vi "TestLightfield.vi"() -> ()   [LabVIEW 2018]
uses:
  <userlib>/LightField Add-in and Automation SDK/Samples/LabVIEW Automation/lightfield-automation-labview/LightField Automation.lvclass
panel:
  out "LightField Error":errorcluster
  in  "Number of Frames":i32=500 min=0 step=1
  in  "On Chip Accumulations":i32=3 min=0 step=1
  in  "stop":bool
  in  "LIGHTFIELD":bool
  in  "Intensifier Gain":i32=100 min=0 max=100 step=1
  in  "Repetitive Gate Delay (us)":dbl=0.25
  in  "Repetitive Gate Width (us)":dbl=400.0 min=0.0 step=0.0001
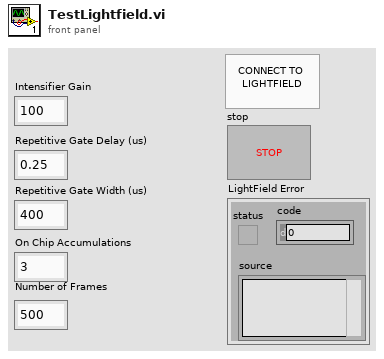
[diagram p1: front panel]
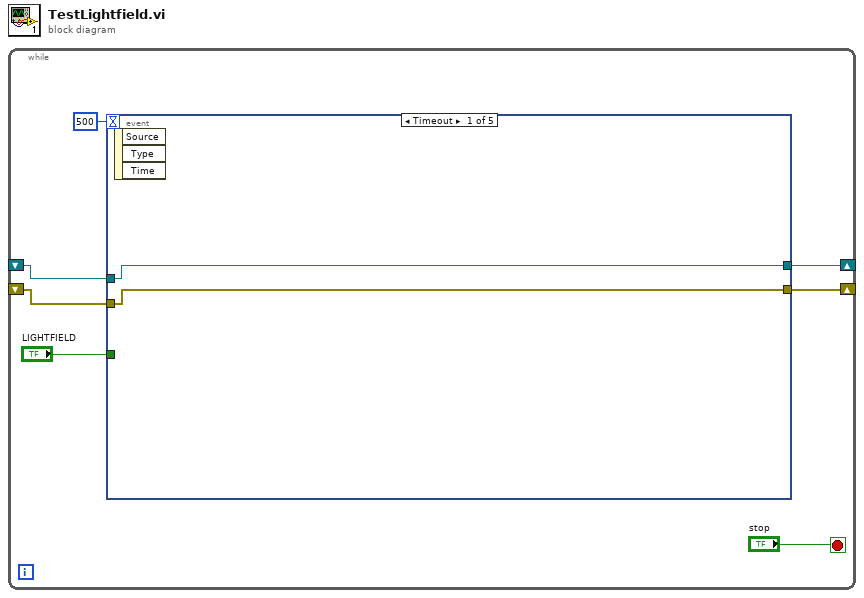
[diagram p0: block diagram]
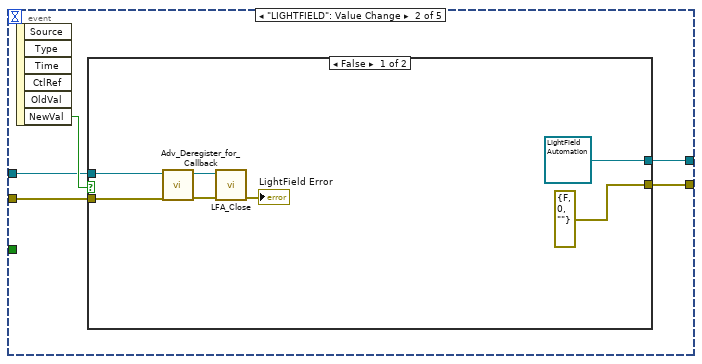
[diagram p2: hidden frame]
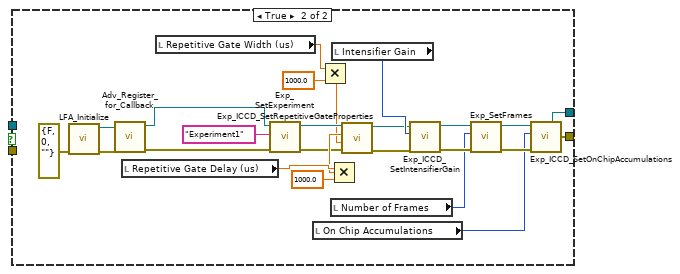
[diagram p3: hidden frame]
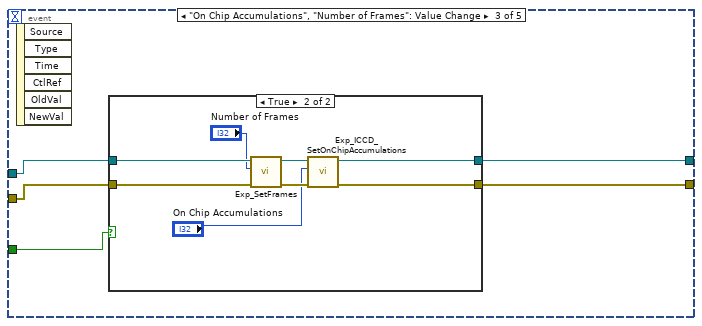
[diagram p4: hidden frame]
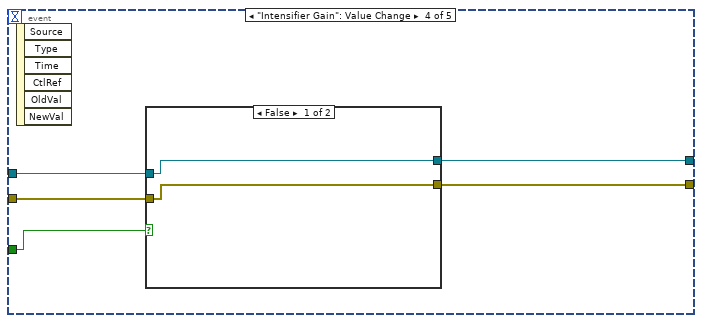
[diagram p6: hidden frame]
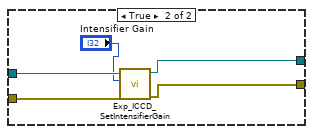
[diagram p7: hidden frame]
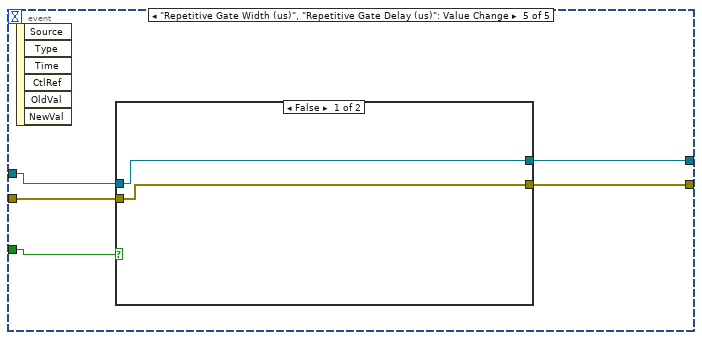
[diagram p8: hidden frame]
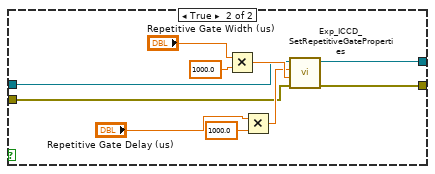
[diagram p9: hidden frame]
diagram:
  n1 = while {
    shift-right: [w4] -> _
    shift-left: _ -> [w7]
    shift-right: [w5] -> _
    shift-left: _ -> [w6]
    stop <- "stop" stop-if-true
    n2 = event shown="[0] Timeout" {
      selector: _ -> [_ _ _ _ _]
      dyn-events: _ -> [_ _ _ _ _]
      timeout: 500 -> [_ _ _ _ _]
      tunnel: w7 -> [w9 w13 w50 w66 w77]
      tunnel: w6 -> [w8 w12 w51 w65 w78]
      tunnel: [w8 w11 w48 w63 w75] -> w5
      tunnel: [w9 w10 w49 w64 w76] -> w4
      tunnel: "LIGHTFIELD" -> [_ _ w47 w62 w74]
      event Timeout {
        n3 = event-data() -> ()  [unwired: 1 in, 3 out]
      }
      event "LIGHTFIELD": Value Change {
        n4 = event-data() -> ("NewVal"=w14:bool)  [unwired: 1 in, 5 out]
        n5 = case shown="False" w14 {
          tunnel: w13 -> [w17 _]
          tunnel: w12 -> [w18 _]
          tunnel: [errorcluster {"status"=FALSE, "code"=0, "source"=""} ("error out") w28] -> w11
          tunnel: [refnum<class "LightField Automation.lvclass"> refnum ("LightField Automation out") w27] -> w10
          frame False {
            n6 = call <userlib>:"Adv_Deregister_for_Callback.vi"("error in (no error)"=w18, "LightField Automation in"=w17) -> ("error out"=w20:errorcluster, "LightField Automation out"=w19:refnum<class "LightField Automation.lvclass">)  [unwired: 8 in]
            n7 = call <userlib>:"LFA_Close.vi"("error in (no error)"=w20, "LightField Automation in"=w19) -> ("error out"=→"LightField Error":errorcluster)  [unwired: 8 in, 1 out]
          }
          frame True {
            n8 = call <userlib>:"LFA_Initialize.vi"("error in (no error)"=errorcluster {"status"=FALSE, "code"=0, "source"=""}) -> ("error out"=w24:errorcluster, "LightField Automation out"=w25:refnum<class "LightField Automation.lvclass">)  [unwired: 9 in]
            n9 = call <userlib>:"Adv_Register_for_Callback.vi"("error in (no error)"=w24, "LightField Automation in"=w25) -> ("error out"=w33:errorcluster, "LightField Automation out"=w32:refnum<class "LightField Automation.lvclass">)  [unwired: 8 in]
            n10 = local read "Repetitive Gate Delay (us)"() -> (w46:dbl)
            n11 = local read "Repetitive Gate Width (us)"() -> (w35:dbl)
            n12 = call <userlib>:"Exp_SetExperiment.vi"("error in (no error)"=w33, "ExperimentName"="Experiment1", "LightField Automation in"=w32) -> ("error out"=w37:errorcluster, "LightField Automation out"=w36:refnum<class "LightField Automation.lvclass">)  [unwired: 7 in]
            n13 = local read "On Chip Accumulations"() -> (w22:i32)
            n14 = Multiply(x=w35, y=1000.0) -> (x*y=w34:dbl)
            n15 = Multiply(x=w46, y=1000.0) -> (x*y=w45:dbl)
            n16 = local read "Number of Frames"() -> (w23:i32)
            n17 = local read "Intensifier Gain"() -> (w40:i32)
            n18 = call <userlib>:"Exp_ICCD_SetRepetitiveGateProperties.vi"("error in (no error)"=w37, "Repetitive Gate Width (ns)"=w34, "Repetitive Gate Delay (ns)"=w45, "LightField Automation in"=w36) -> ("error out"=w38:errorcluster, "LightField Automation out"=w39:refnum<class "LightField Automation.lvclass">)  [unwired: 6 in]
            n19 = call <userlib>:"Exp_ICCD_SetIntensifierGain.vi"("error in (no error)"=w38, "Intensifier Gain"=w40, "LightField Automation in"=w39) -> ("error out"=w41:errorcluster, "LightField Automation out"=w42:refnum<class "LightField Automation.lvclass">)  [unwired: 7 in]
            n20 = call <userlib>:"Exp_SetFrames.vi"("error in (no error)"=w41, "Number of Frames"=w23, "LightField Automation in"=w42) -> ("error out"=w44:errorcluster, "LightField Automation out"=w43:refnum<class "LightField Automation.lvclass">)  [unwired: 7 in]
            n21 = call <userlib>:"Exp_ICCD_SetOnChipAccumulations.vi"("error in (no error)"=w44, "On Chip Accumulations"=w22, "LightField Automation in"=w43) -> ("error out"=w28:errorcluster, "LightField Automation out"=w27:refnum<class "LightField Automation.lvclass">)  [unwired: 7 in]
          }
        }
      }
      event "On Chip Accumulations", "Number of Frames": Value Change {
        n22 = event-data() -> ()  [unwired: 1 in, 6 out]
        n23 = case shown="True" w47 {
          tunnel: w51 -> [w52 w59]
          tunnel: w50 -> [w53 w58]
          tunnel: [w53 w57] -> w49
          tunnel: [w52 w56] -> w48
          frame False {
          }
          frame True {
            n24 = call <userlib>:"Exp_SetFrames.vi"("error in (no error)"=w59, "Number of Frames"="Number of Frames", "LightField Automation in"=w58) -> ("error out"=w60:errorcluster, "LightField Automation out"=w61:refnum<class "LightField Automation.lvclass">)  [unwired: 7 in]
            n25 = call <userlib>:"Exp_ICCD_SetOnChipAccumulations.vi"("error in (no error)"=w60, "On Chip Accumulations"="On Chip Accumulations", "LightField Automation in"=w61) -> ("error out"=w56:errorcluster, "LightField Automation out"=w57:refnum<class "LightField Automation.lvclass">)  [unwired: 7 in]
          }
        }
      }
      event "Intensifier Gain": Value Change {
        n26 = event-data() -> ()  [unwired: 1 in, 6 out]
        n27 = case shown="False" w62 {
          tunnel: w66 -> [w68 w73]
          tunnel: w65 -> [w67 w72]
          tunnel: [w68 w70] -> w64
          tunnel: [w67 w69] -> w63
          frame False {
          }
          frame True {
            n28 = call <userlib>:"Exp_ICCD_SetIntensifierGain.vi"("error in (no error)"=w72, "Intensifier Gain"="Intensifier Gain", "LightField Automation in"=w73) -> ("error out"=w69:errorcluster, "LightField Automation out"=w70:refnum<class "LightField Automation.lvclass">)  [unwired: 7 in]
          }
        }
      }
      event "Repetitive Gate Width (us)", "Repetitive Gate Delay (us)": Value Change {
        n29 = event-data() -> ()  [unwired: 1 in, 6 out]
        n30 = case shown="False" w74 {
          tunnel: w78 -> [w79 w84]
          tunnel: w77 -> [w80 w83]
          tunnel: [w80 w82] -> w76
          tunnel: [w79 w81] -> w75
          frame False {
          }
          frame True {
            n31 = Multiply(x="Repetitive Gate Width (us)", y=1000.0) -> (x*y=w89:dbl)
            n32 = Multiply(x="Repetitive Gate Delay (us)", y=1000.0) -> (x*y=w87:dbl)
            n33 = call <userlib>:"Exp_ICCD_SetRepetitiveGateProperties.vi"("error in (no error)"=w84, "Repetitive Gate Width (ns)"=w89, "Repetitive Gate Delay (ns)"=w87, "LightField Automation in"=w83) -> ("error out"=w81:errorcluster, "LightField Automation out"=w82:refnum<class "LightField Automation.lvclass">)  [unwired: 6 in]
          }
        }
      }
    }
  }
